vi "ClarkeTest.vi"(7 "Resources":T1, 9 "C":sgl, 10 "B":sgl, 11 "A":sgl) -> (2 "beta":sgl, 3 "alpha":sgl)   [LabVIEW 2016]
uses:
  Adder/Adder.lvclass
  Subtractor/Subtractor.lvclass
  Multiplier/Multiplier.lvclass
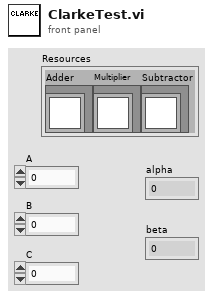
[diagram p1: front panel]
types:
  T1 = cluster{"Adder":refnum<class "Adder.lvclass">, "Multiplier":refnum<class "Multiplier.lvclass">, "Subtractor":refnum<class "Subtractor.lvclass">}
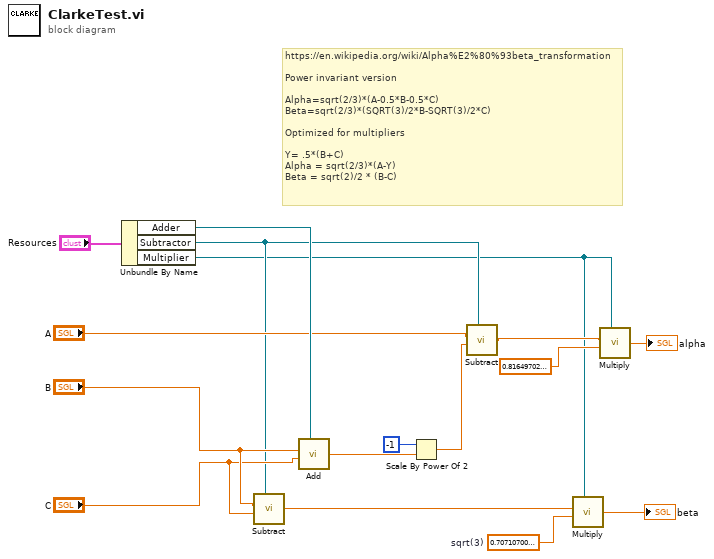
[diagram p0: block diagram]
diagram:
  w4 = sgl 0.707107  # sqrt(3)
  # "https://en.wikipedia.org/wiki/Alpha%E2%80%93beta_transformation\n\nPower invariant version\n\nAlpha=sqrt(2/3)*(A-0.5*B-0.5*C)\nBeta=sqrt(2/3)*(SQRT(3)/2*B-SQRT(3)/2*C)\n\nOptimized for multipliers\n\nY= .5*(B+C)\nAlpha = sqrt(2/3)*(A-Y)\nBeta = sqrt(2)/2 * (B-C)"
  n1 = Unbundle By Name("Resources") -> ("Adder"=w13:refnum<class "Adder.lvclass">, "Subtractor"=w8:refnum<class "Subtractor.lvclass">, "Multiplier"=w2:refnum<class "Multiplier.lvclass">)
  n2 = call-dynamic "Subtract.vi"("x"="B", "y"="C", "Subtractor"=w8) -> ("x-y"=w3:sgl)  [unwired: 4 in]
  n3 = call-dynamic "Add.vi"("x"="B", "y"="C", "Adder"=w13) -> ("x+y"=w14:sgl)  [unwired: 4 in]
  n4 = Scale By Power Of 2(n=i16 -1, x=w14) -> (x*2^n=w9:sgl)
  n5 = call-dynamic "Subtract.vi"("x"="A", "y"=w9, "Subtractor"=w8) -> ("x-y"=w6:sgl)  [unwired: 4 in]
  n6 = call-dynamic "Multiply.vi"("x"=w3, "y"=w4, "Multiplier"=w2) -> ("x*y"=→"beta":sgl)  [unwired: 4 in]
  n7 = call-dynamic "Multiply.vi"("x"=w6, "y"=sgl 0.816497, "Multiplier"=w2) -> ("x*y"=→"alpha":sgl)  [unwired: 4 in]
